vi "decimate array.vi"(10 "decimation factor":dbl, 11 "input array":dbl[](array[numeric])) -> (3 "decimated array":dbl[](array[numeric]))   [LabVIEW 2014]
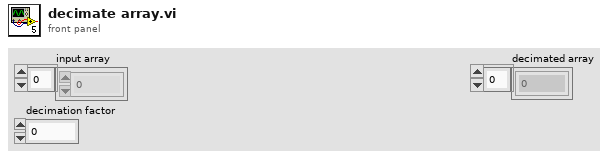
[diagram p1: front panel]
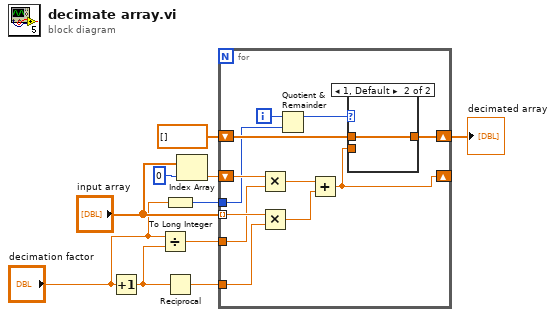
[diagram p0: block diagram]
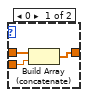
[diagram p2: hidden frame]
diagram:
  n1 = Increment(x="decimation factor") -> (x+1=w10:dbl)
  n2 = Divide(x="decimation factor", y=w10) -> (x/y=w7:dbl)
  n3 = To Long Integer(number="decimation factor") -> (32bit integer=w4:i32)
  n4 = Reciprocal(x=w10) -> (1/x=w6:dbl)
  n5 = Index Array(array="input array", index=0) -> (element=w9:dbl)
  n6 = for {
    tunnel: "input array" -> [w21] mode=indexing
    tunnel: w6 -> [w22]
    tunnel: w7 -> [w20]
    shift-right: [w14] -> _
    shift-left: w9 -> [w19]
    tunnel: w4 -> [w11]
    shift-right: [w12] -> w1
    shift-left: dbl[] [] -> [w13]
    i -> [w16]
    n7 = Multiply(x=w19, y=w20) -> (x*y=w18:dbl)
    n8 = Multiply(x=w21, y=w22) -> (x*y=w17:dbl)
    n9 = Quotient & Remainder(x=w16, y=w11) -> (x-y*floor(x/y)=w15:i32)  [unwired: 1 out]
    n10 = Add(x=w18, y=w17) -> (x+y=w14:dbl)
    n11 = case shown="1, Default" w15 {
      tunnel: w14 -> [w25 _]
      tunnel: w13 -> [w24 w26]
      tunnel: [w23 w26] -> w12
      frame 0 {
        n12 = Build Array (concatenate)(w24, w25) -> (w23:dbl[])
      }
      frame 1, Default {
      }
    }
  }
  "decimated array" <- w1
